vi "Result.vi"() -> (3 "out Result":refnum<class "Result.lvclass">)   [LabVIEW 2024, in "Result.lvclass"]
uses:
  Result.lvclass
  Result.lvclass/Result.ctl
panel:
  in  "String":string
  in  "Numeric":dbl
  in  "Result.lvclass":refnum<class "Result.lvclass">
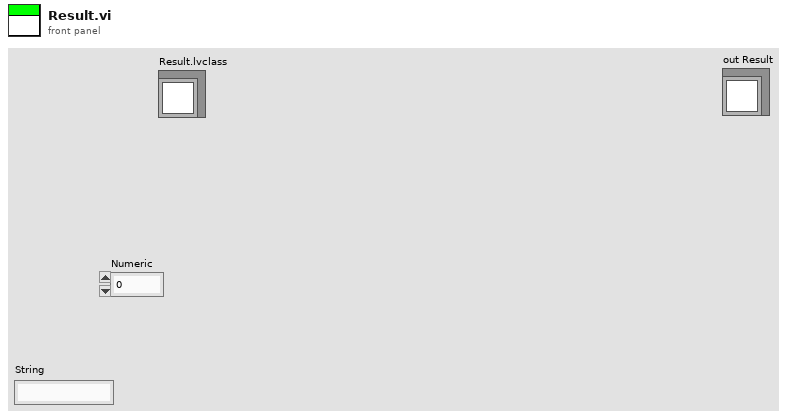
[diagram p1: front panel]
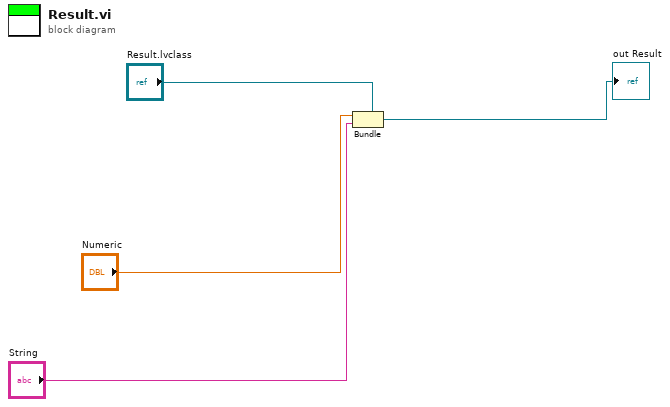
[diagram p0: block diagram]
diagram:
  n1 = Bundle(cluster="Result.lvclass", "Numeric", "String") -> (→"out Result":refnum<class "Result.lvclass">)
